vi "Creators Status Created Events.vi"(11 "Base Event jettl in":refnum<class "Base Event jettl.lvclass">) -> (0 "Created Event Count":i32, 1 "Created Event Aliases":string[](array[string]), 2 "Created Event Exist?":bool, 3 "Base Event jettl out":refnum<class "Base Event jettl.lvclass">)   [LabVIEW 2021, in "jettl.lvlib" / "Base Event jettl.lvlib" / "Base Event jettl.lvclass"]
uses:
  Base Event jettl.lvclass
  C:/git/jettl/src/jettl/jettl/jettl.lvclass
  Base Event jettl.lvclass/Base Event jettl.ctl
  Queue Mailbox/Queue Mailbox.lvlib
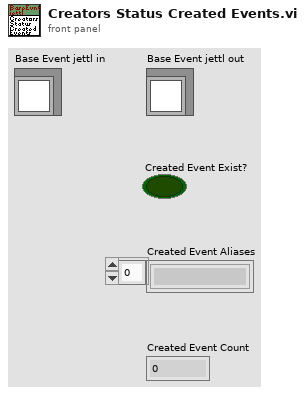
[diagram p1: front panel]
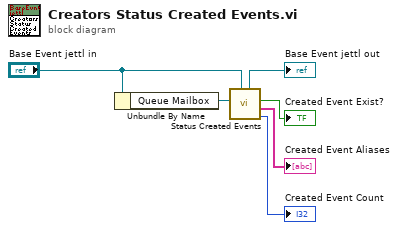
[diagram p0: block diagram]
diagram:
  n1 = Unbundle By Name("Base Event jettl in") -> ("Queue Mailbox"=w5:refnum<data-value>)
  n2 = call "Status Created Events.vi"("jettl in"="Base Event jettl in", "Queue Mailbox"=w5) -> ("Created Event Count"=→"Created Event Count":i32, "Created Event Aliases"=→"Created Event Aliases":string[], "Created Event Exist?"=→"Created Event Exist?":bool, "jettl out"=→"Base Event jettl out":refnum<class "Base Event jettl.lvclass">)  [unwired: 6 in]
